vi "SIM Registry Update Vector Widths.vi"(5 "Output Width":i32, 6 "Node Headers":T1[](array[typedef]), 7 "Input Width":i32, 10 "Block Idx":i32) -> (2 "Block Idx Out":i32, 4 "Node Headers Out":T1[](array[typedef]))   [LabVIEW 2020]
uses:
  <vilib>/Simulation/Implementation/Shared/SIM Registry.llb/SIM Registry Node Header.ctl
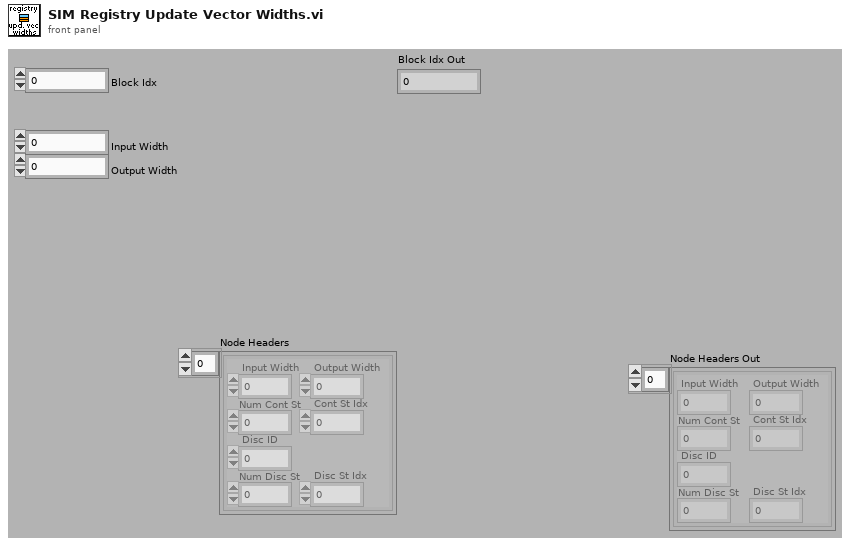
[diagram p1: front panel]
types:
  T1 = typedef "SIM Registry Node Header.ctl" = cluster{"Input Width":i32, "Disc ID":i32, "Num Cont St":i32, "Cont St Idx":i32, "Num Disc St":i32, "Disc St Idx":i32, "Output Width":i32}
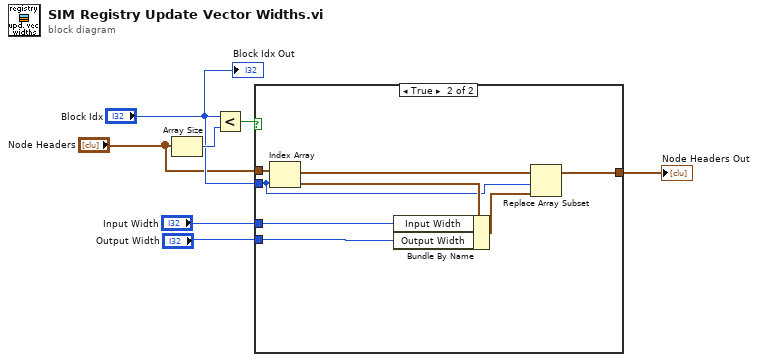
[diagram p0: block diagram]
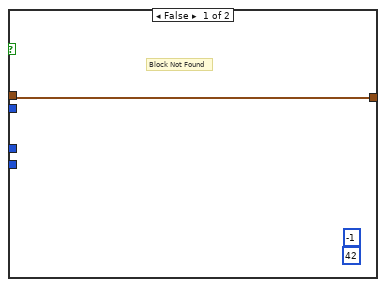
[diagram p2: hidden frame]
diagram:
  n1 = Array Size(array="Node Headers") -> (size(s)=w7:i32)
  n2 = Less?(x="Block Idx", y=w7) -> (x < y?=w6:bool)
  n3 = case shown="True" w6 {
    tunnel: "Node Headers" -> [w8 w14]
    tunnel: "Block Idx" -> [_ w12]
    tunnel: "Output Width" -> [_ w10]
    tunnel: [w8 w11] -> w2
    tunnel: "Input Width" -> [_ w9]
    frame False {
      (unwired) 42 ("error out")
      (unwired) -1 ("state idx")
      # "Block Not Found"
    }
    frame True {
      n4 = Index Array(array=w14, index=w12) -> (element=w15:T1)
      n5 = Bundle By Name(cluster=w15, "Input Width"=w9, "Output Width"=w10) -> (w13:T1)
      n6 = Replace Array Subset(array=w14, new element=w13, index=w12) -> (w11:T1[])
    }
  }
  "Node Headers Out" <- w2
  "Block Idx Out" <- "Block Idx"
